vi "unpack frame.vi"(9 "timestamp in":u64 format="%x", 10 "frame":u8[](array[numeric]) format="%x", 11 "status in":u32 format="%x") -> (0 "timestamp out":u64, 1 "data":u8[](array[numeric]) format="%x", 2 "id":u32 format="%x", 3 "status out":u32 format="%x", 4 "message type":T5, 5 "queue empty?":bool, 6 "ecc register":T1)   [LabVIEW 2024, in "atsj peakcan basic.lvlib"]
uses:
  atsj peakcan basic.lvlib
  message type.ctl
  ecc register.ctl
  ecc register error code.ctl
  ecc register direction.ctl
  ecc register segment.ctl
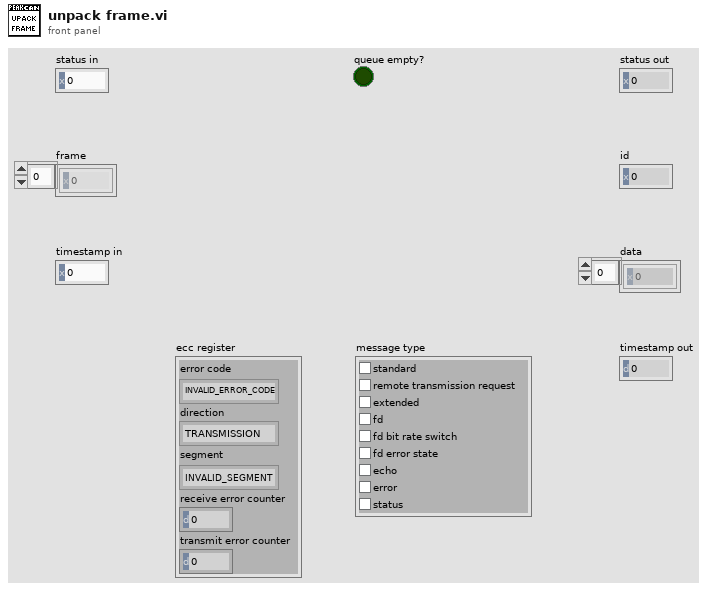
[diagram p1: front panel]
types:
  T1 = typedef "atsj peakcan basic.lvlib/ecc register.ctl" = cluster{"error code":T2, "direction":T3, "segment":T4, "receive error counter":u8, "transmit error counter":u8}
  T2 = typedef "atsj peakcan basic.lvlib/ecc register error code.ctl" = enum8{"INVALID_ERROR_CODE", "COUNTERS_UPDATE", "BIT_ERROR", "FORM_ERROR", "STUFF_ERROR", "OTHER_ERROR"}
  T3 = typedef "atsj peakcan basic.lvlib/ecc register direction.ctl" = enum16{"TRANSMISSION", "RECEPTION"}
  T4 = typedef "atsj peakcan basic.lvlib/ecc register segment.ctl" = enum8{"INVALID_SEGMENT", "ID_28_TO_ID_21", "START_OF_FRAME", "BIT_SRTR", "BIT_IDE", "ID_20_TO_ID_18", "ID_17_TO_ID_13", "CRC_SEQUENCE", "RESERVED_BIT_0", "DATA_FIELD", "DATA_LENGTH_CODE", "BIT_RTR", "RESERVED_BIT_1", "ID_4_TO_ID_0", "ID_12_TO_ID_5", "ACTIVE_ERROR_FLAG", "INTERMISSION", "TOLERATE_DOMINANT_BITS", "ERROR_DELIMITER", "CRC_DELIMITER", "ACKNOWLEDGE_SLOT", "END_OF_FRAME", "ACKNOWLEDGE_LIMITER", "OVERLOAD_FLAG"}
  T5 = typedef "atsj peakcan basic.lvlib/message type.ctl" = cluster{"standard":bool, "remote transmission request ":bool, "extended":bool, "fd":bool, "fd bit rate switch":bool, "fd error state":bool, "echo":bool, "error":bool, "status":bool}
  T6 = cluster{"Boolean array[0]":bool, "Boolean array[1]":bool, "Boolean array[2]":bool, "Boolean array[3]":bool, "Boolean array[4]":bool, "Boolean array[5]":bool, "Boolean array[6]":bool, "Boolean array[7]":bool, "Boolean array[8]":bool}
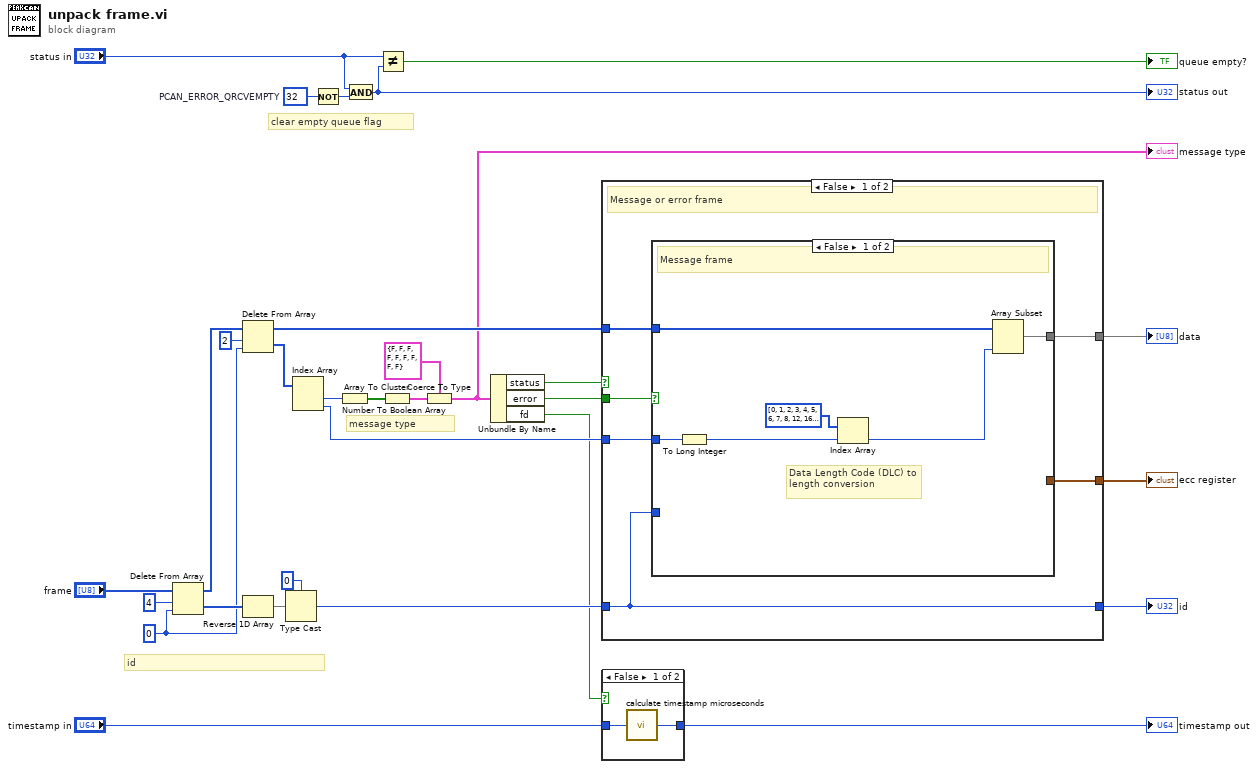
[diagram p0: block diagram]
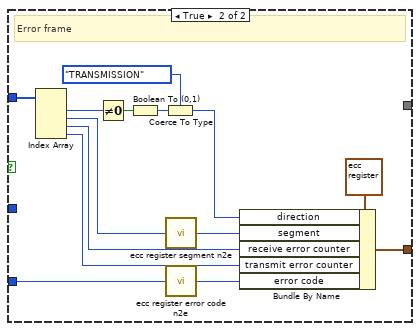
[diagram p3: hidden frame]
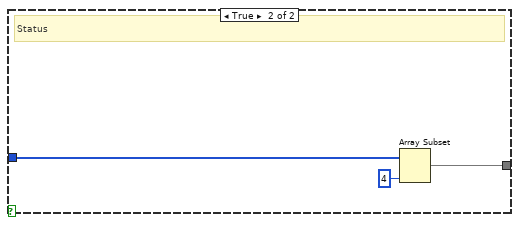
[diagram p4: hidden frame]
diagram:
  w2 = u32 32  # PCAN_ERROR_QRCVEMPTY
  w25 = 0
  # "clear empty queue flag"
  # "message type"
  # "id"
  n1 = Delete From Array(array="frame", length=4, index=w25) -> (deleted portion=w29:u8[], array with subset deleted=w26:u8[])
  n2 = Delete From Array(array=w26, length=2, index=w25) -> (deleted portion=w23:u8[], array with subset deleted=w14:u8[])
  n3 = Reverse 1D Array(array=w29) -> (reversed array=w28:u8[])
  n4 = Type Cast(type=u32 0, x=w28) -> (*(type *) &x=w12:u32)
  n5 = Index Array(array=w23) -> (element #1=w22:u8, element #2=w15:u8)  [unwired: 2 in]
  n6 = Not(x=w2) -> (.not. x?=w6:u32)
  n7 = Number To Boolean Array(number=w22) -> (Boolean array=w21:bool[])
  n8 = And(x="status in", y=w6) -> (x .and. y?=w3:u32)
  "status out" <- w3
  n9 = Not Equal?(x="status in", y=w3) -> (x != y?=→"queue empty?":bool)
  n10 = Array To Cluster(array=w21) -> (cluster=w20:T6)
  n11 = Coerce To Type(0:w20, 1:T5 {"standard"=FALSE, "remote transmission request "=FALSE, "extended"=FALSE, "fd"=FALSE, "fd bit rate switch"=FALSE, "fd error state"=FALSE, "echo"=FALSE, "error"=FALSE, "status"=FALSE}) -> (2:w10:T5)
  "message type" <- w10
  n12 = Unbundle By Name(w10) -> ("status"=w17:bool, "error"=w16:bool, "fd"=w9:bool)
  n13 = case shown="False" w17 {
    tunnel: w16 -> [w36 _]
    tunnel: w15 -> [w35 _]
    tunnel: w14 -> [w34 w59]
    tunnel: [w33 w57] -> w13
    tunnel: w12 -> [w32 _]
    tunnel: [w32 _] -> w11
    tunnel: [w31 _] -> w1
    frame False {
      # "Message or error frame"
      n14 = case shown="False" w36 {
        tunnel: w35 -> [w41 _]
        tunnel: w34 -> [w40 w51]
        tunnel: [w39 _] -> w33
        tunnel: w32 -> [_ w52]
        tunnel: [_ w43] -> w31
        frame False {
          # "Data Length Code (DLC) to length conversion"
          # "Message frame"
          n15 = To Long Integer(number=w41) -> (32bit integer=w38:i32)
          n16 = Index Array(array=i32[] [0, 1, 2, 3, 4, 5, 6, 7, 8, 12, 16, 20, 24, 32, 48, 64], index=w38) -> (element=w42:i32)
          n17 = Array Subset(array=w40, length=w42) -> (w39:u8[])  [unwired: 1 in]
        }
        frame True {
          # "Error frame"
          n18 = Index Array(array=w51) -> (element #1=w50:u8, element #2=w49:u8, element #3=w46:u8, element #4=w45:u8)  [unwired: 4 in]
          n19 = Not Equal To 0?(x=w50) -> (x != 0?=w55:bool)
          n20 = Boolean To (0,1)(Boolean=w55) -> (0, 1=w56:i16)
          n21 = Coerce To Type(0:w56, 1:ecc_register_direction."TRANSMISSION") -> (2:w48:T3)
          n22 = call "ecc register segment n2e.vi"("number"=w49) -> ("enum"=w47:T4)
          n23 = call "ecc register error code n2e.vi"("number"=w52) -> ("enum"=w44:T2)
          n24 = Bundle By Name(cluster=T1 {"error code"=enum."INVALID_ERROR_CODE", "direction"=enum."TRANSMISSION", "segment"=enum."INVALID_SEGMENT", "receive error counter"=0, "transmit error counter"=0}, "direction"=w48, "segment"=w47, "receive error counter"=w46, "transmit error counter"=w45, "error code"=w44) -> (w43:T1)
        }
      }
    }
    frame True {
      # "Status"
      n25 = Array Subset(array=w59, length=4) -> (w57:u8[])  [unwired: 1 in]
    }
  }
  "id" <- w11
  "data" <- w13
  "ecc register" <- w1
  n26 = case shown="False" w9 {
    tunnel: [w61 w62] -> w8
    tunnel: "timestamp in" -> [w60 w62]
    frame False {
      n27 = call "calculate timestamp microseconds.vi"("timestamp in"=w60) -> ("timestamp out"=w61:u64)
    }
    frame True {
    }
  }
  "timestamp out" <- w8
